vi "APT_Error.vi"(1 "Return Code":i32, 2 "error in (no error)":errorcluster) -> (0 "error out":errorcluster)   [LabVIEW 2010]
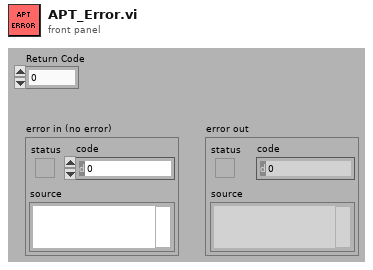
[diagram p1: front panel]
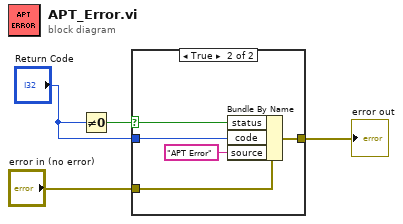
[diagram p0: block diagram]
diagram:
  n1 = Not Equal To 0?(x="Return Code") -> (x != 0?=w3:bool)
  n2 = case shown="True" w3 {
    selector: w3 -> [_ w9]
    tunnel: "Return Code" -> [_ w8]
    tunnel: "error in (no error)" -> [w5 w10]
    tunnel: [w5 w6] -> w1
    frame False {
    }
    frame True {
      n3 = Bundle By Name(cluster=w10, "status"=w9, "code"=w8, "source"="APT Error") -> (w6:errorcluster)
    }
  }
  "error out" <- w1
